vi "niDTS BT LE Rx Test Get Default Parameters.vi"(0 "Dummy Test Handle In":T1, 11 "error in (no error)":errorcluster) -> (4 "Dummy Test Handle Out 2":T1, 8 "BDR Tx Parameters":T2={"Channel"=1, "Tx Power (dBm)"=0.0, "External Attenuation (dB)"=0.0, "Payload Data"=enum."00001111", "Carrier Mode"=enum."Burst", "Number of Packets"=4, "Corrupt Alternate CRC"=FALSE, "Dirty Tx"=FALSE, "Payload Header"={"Length (-1 AutoSet Max)"=0}, "Trigger"={"TriggerEdge"=enum."RISing", "TriggerSource"=enum."IMMediate", "TriggerDelay (sec)"=0.0, "TriggerTimeout (sec)"=0.0}}, 15 "error out":errorcluster)   [LabVIEW 2014, in "niDTS BT.lvlib"]
uses:
  niDTS BT.lvlib
  Includes/niDTS BT LE Rx Test INC Parameters.ctl
  Tx Test/Includes/niDTS BT Tx Test INC BD Payload Data.ctl
  Rx Test/Includes/niDTS BT Rx Test INC Carrier Mode.ctl
  Rx Test/Includes/niDTS BT Rx Test INC LE Payload Length.ctl
  Includes/niDTS BT DUT INC SG Trigger.ctl
  BDR Tx Test/Includes/niDTS BT Rx Test INC Handle.ctl
  Rx Test/Objects/BASE_class/niDTS BT Rx Test.lvclass
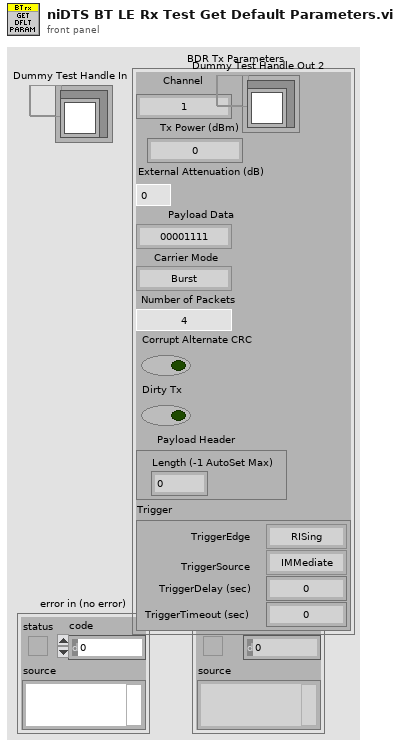
[diagram p1: front panel]
types:
  T1 = typedef "niDTS BT.lvlib/niDTS BT Rx Test INC Handle.ctl" = refnum<data-value>
  T2 = typedef "niDTS BT.lvlib/niDTS BT LE Rx Test INC Parameters.ctl" = cluster{"Channel":i32, "Tx Power (dBm)":dbl, "External Attenuation (dB)":dbl, "Payload Data":T3, "Carrier Mode":T4, "Number of Packets":i32, "Corrupt Alternate CRC":bool, "Dirty Tx":bool, "Payload Header":T5, "Trigger":T6}
  T3 = typedef "niDTS BT.lvlib/niDTS BT Tx Test INC BD Payload Data.ctl" = enum16{"0", "1", "01", "00001111", "PN9", "AUTO"}
  T4 = typedef "niDTS BT.lvlib/niDTS BT Rx Test INC Carrier Mode.ctl" = enum16{"Burst", "Continuous"}
  T5 = typedef "niDTS BT.lvlib/niDTS BT Rx Test INC LE Payload Length.ctl" = cluster{"Length (-1 AutoSet Max)":i32}
  T6 = typedef "niDTS BT.lvlib/niDTS BT DUT INC SG Trigger.ctl" = cluster{"TriggerEdge":enum16{"RISing", "FALLing"}, "TriggerSource":enum16{"IMMediate", "PFI 0", "PFI 1", "RTSI 0", "RTSI 1", "RTSI 2", "RTSI 3", "RTSI 4", "RTSI 5", "RTSI 6", "RTSI 7", "PXI STAR", "Software"}, "TriggerDelay (sec)":dbl, "TriggerTimeout (sec)":dbl}
  T7 = typedef "niDTS BT.lvlib/niDTS BT Rx Test INC Parameters.ctl" = cluster{"Channel":i32, "Dut Tx Power":dbl, "External Attenuation (dB)":dbl[], "Data Rate":enum16{"1", "2", "3"}, "Packet type":T8, "Payload Data":T3, "Carrier Mode":T4, "Number of Packets":i32, "Report Period (ms)":dbl, "BD ADDRESS":i64, "Dirty Tx":bool, "Corrupt Alternate CRC":bool, "Packet Header":T9, "Payload Header":T10, "Trigger":T6}
  T8 = typedef "niDTS BT.lvlib/niDTS BT INC Packet Type.ctl" = enum16{"NULL", "POLL", "FHS", "DM1", "DH1", "HV1", "HV2", "HV3", "EV3", "DV", "AUX1", "DM3", "DH3", "EV4", "EV5", "DM5", "DH5", "LE-TP"}
  T9 = typedef "niDTS BT.lvlib/niDTS BT Rx Test INC Packet Header.ctl" = cluster{"LT Address":i8, "Flow":i8, "ARQN":enum16{"NAK", "ACK"}, "Sequence Bit":i8}
  T10 = typedef "niDTS BT.lvlib/niDTS BT Rx Test INC Payload Header.ctl" = cluster{"LCh":i32, "HeaderFlowControlBit":bool, "Length (-1 AutoSet Max)":i32}
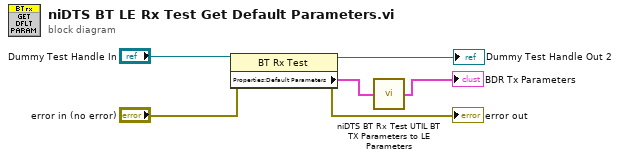
[diagram p0: block diagram]
diagram:
  n1 = property class="BT Rx Test"(reference="Dummy Test Handle In", error in="error in (no error)") -> (reference out=→"Dummy Test Handle Out 2":T1, error out=→"error out":errorcluster, "Properties:Default Parameters"=w2:T7)
  n2 = call "niDTS BT Rx Test UTIL BT TX Parameters to LE Parameters.vi"("BT Tx Parameters"=w2) -> ("BT BDR Parameters"=→"BDR Tx Parameters":T2)  [unwired: 14 in]
